vi "RTM - Tx Create Channels.vi"(6 "NumberOfInstances":u32, 7 "AppendToChannels":bool, 8 "error in (no error)":errorcluster, 9 "Descriptions":string[](array[string]), 10 "Channel Configuration":string[][](array[string]), 11 "Node Ptr":T1 format="%.0x") -> (0 "error out":errorcluster, 1 "ChannelPaths":string[](array[string]), 2 "ChannelNames":string[](array[string]), 4 "ChannelDataTypes":string[](array[string]), 5 "ChannelRefs":T1[](array[typedef]) format="%.0x")   [LabVIEW 2019, in "UDP-Custom-Device System Explorer.lvlib"]
uses:
  UDP-Custom-Device System Explorer.lvlib
  <vilib>/NI VeriStand/Custom Device API/Custom Device Item Ref.ctl
  <vilib>/NI VeriStand/Custom Device API/Custom Device Channel.ctl
  <vilib>/NI VeriStand/Custom Device API/Custom Device Channel Type.ctl
  Shared/Constants.vi
  <vilib>/NI VeriStand/Custom Device API/Custom Device API.lvlib
  Shared/UDP-Custom-Device Shared.lvlib
  Property Accessors/Tx Channel Section Accessors.lvlib
  Property Accessors/Tx Channel Accessors.lvlib
panel:
  out "ExistingChannels":string[](array[string])
  out "Dependent Node Refs":T1[](array[typedef]) format="%.0x"
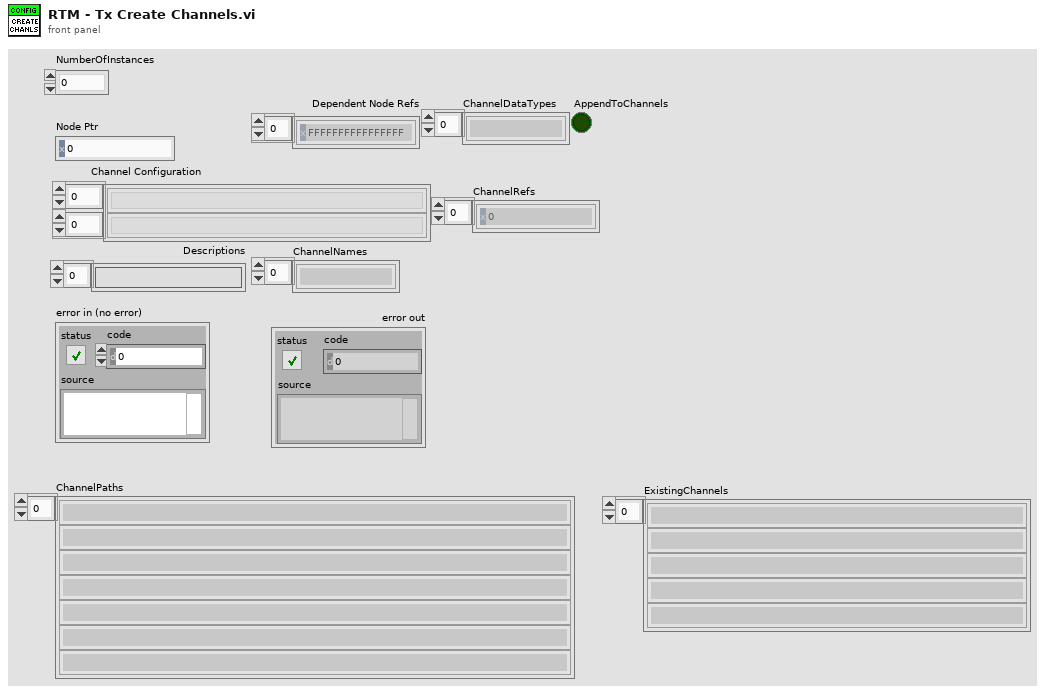
[diagram p1: front panel]
types:
  T1 = typedef "Custom Device API.lvlib/Custom Device Item Ref.ctl" = u64
  T2 = typedef "Custom Device API.lvlib/Custom Device Channel.ctl" = cluster{"Type":T3, "Units":string, "Default Value":dbl, "Faultable":bool, "Scalable":bool}
  T3 = typedef "Custom Device API.lvlib/Custom Device Channel Type.ctl" = enum16{"Input", "Output"}
  T4 = typedef "UDP-Custom-Device Shared.lvlib/Shared - Channel Data Type.ctl" = enum16{"Boolean", "Single", "Double", "I8", "I16", "I32", "I64", "U8", "U16", "U32", "U64"}
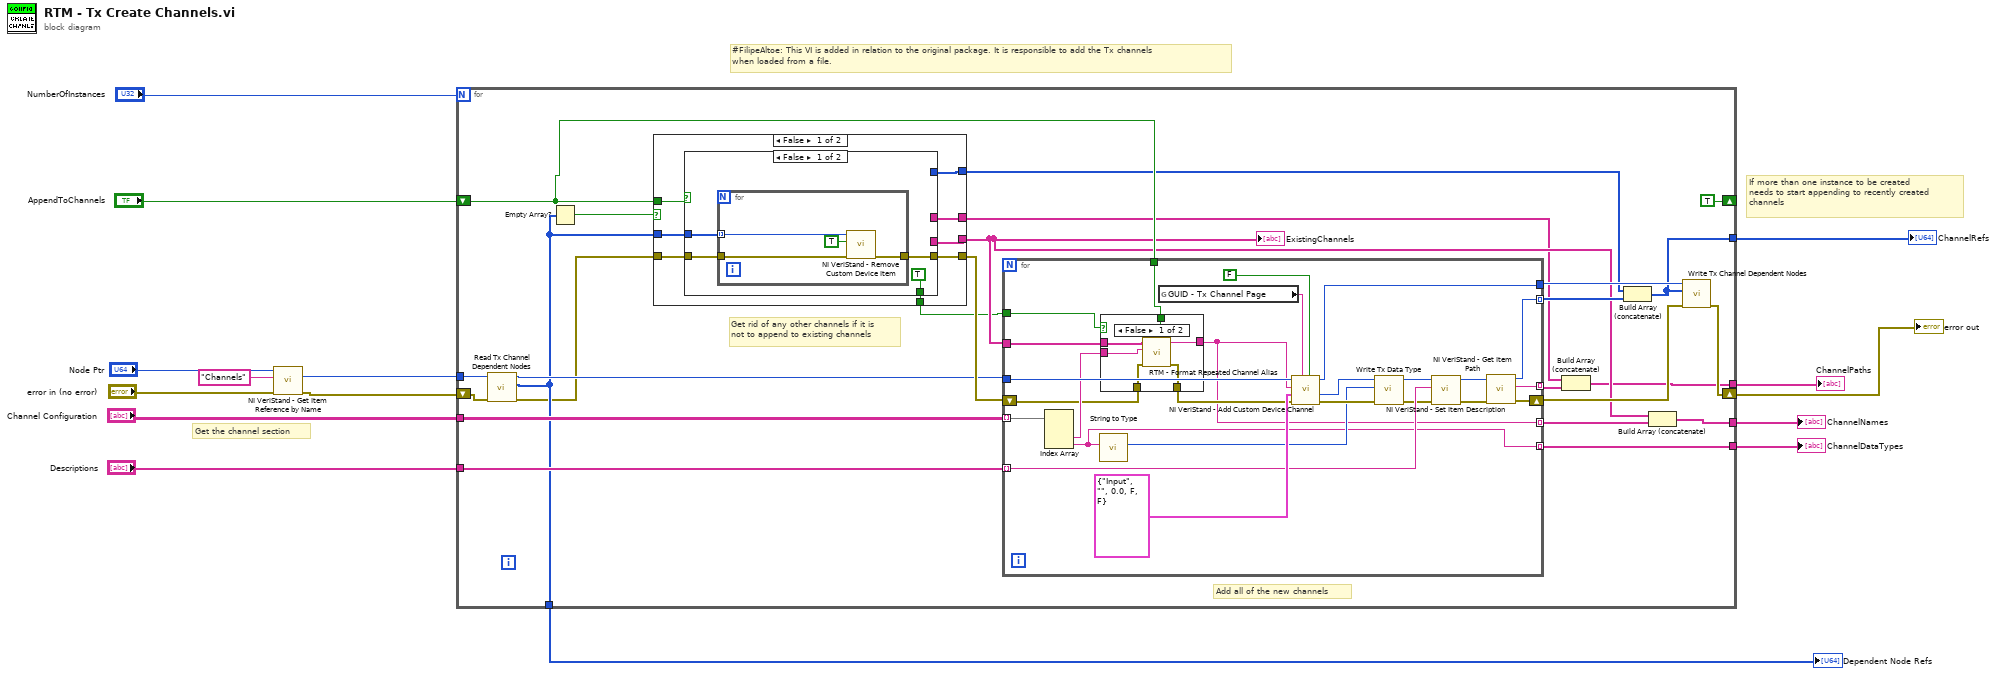
[diagram p0: block diagram]
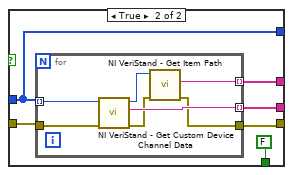
[diagram p3: hidden frame]
diagram:
  # "If more than one instance to be created\nneeds to start appending to recently created\nchannels"
  # "#FilipeAltoe: This VI is added in relation to the original package. It is responsible to add the Tx channels\nwhen loaded from a file."
  # "Get the channel section"
  n1 = call <vilib>:"NI VeriStand - Get Item Reference by Name.vi"("error in (no error)"="error in (no error)", "Item Name"="Channels" ("Section Name"), "Parent Ref in"="Node Ptr") -> ("error out"=w9:errorcluster, "Item Ref"=w3:T1)  [unwired: 5 in, 2 out]
  n2 = for {
    N: "NumberOfInstances" -> [_]
    tunnel: "Descriptions" -> [w39]
    tunnel: "Channel Configuration" -> [w38]
    tunnel: [w36] -> w10
    tunnel: [w25] -> w8
    tunnel: [w22] -> w6
    tunnel: [w18] -> w5
    tunnel: [w20] -> w4
    tunnel: w3 -> [w27]
    shift-right: [w31] -> w7
    shift-left: w9 -> [w35]
    shift-right: [TRUE ("AppendToChannels")] -> _
    shift-left: "AppendToChannels" -> [w26]
    # "Add all of the new channels"
    # "Get rid of any other channels if it is\nnot to append to existing channels"
    n3 = call "Read Tx Channel Dependent Nodes.vi"("error in (no error)"=w35, "Node Ptr"=w27) -> ("error out"=w34:errorcluster, "Dependent Node Refs"=w36:T1[], "Node Ptr out"=w37:T1)  [unwired: 7 in]
    n4 = Empty Array?(array=w36) -> (empty?=w23:bool)
    n5 = case shown="False" w23 {
      selector: w23 -> [_ w103]
      tunnel: [w81 w104] -> w40
      tunnel: w34 -> [w80 w104]
      tunnel: w36 -> [w79 _]
      tunnel: [w77 _] -> w21
      tunnel: w26 -> [w78 _]
      tunnel: [w76 _] -> w24
      tunnel: [w75 _] -> w19
      tunnel: [w74 w103] -> w17
      frame False {
        n6 = case shown="False" w78 {
          tunnel: [w85 w93] -> w81
          tunnel: w80 -> [w84 w95]
          tunnel: w79 -> [w83 w92]
          tunnel: [_ w94] -> w77
          tunnel: [_ w92] -> w76
          tunnel: [_ w91] -> w75
          tunnel: [TRUE FALSE] -> w74
          frame False {
            n7 = for {
              tunnel: w83 -> [w86] mode=indexing
              tunnel: [w88] -> w85
              tunnel: w84 -> [w87]
              n8 = call <vilib>:"NI VeriStand - Remove Custom Device Item.vi"("error in (no error)"=w87, "Force Delete (F)"=TRUE, "Item Ref in"=w86) -> ("error out"=w88:errorcluster)  [unwired: 7 in, 1 out]
            }
          }
          frame True {
            n9 = for {
              tunnel: w92 -> [w102] mode=indexing
              tunnel: [w98] -> w93
              tunnel: w95 -> [w101]
              tunnel: [w100] -> w94 mode=indexing
              tunnel: [w96] -> w91 mode=indexing
              n10 = call <vilib>:"NI VeriStand - Get Custom Device Channel Data.vi"("error in (no error)"=w101, "Channel Ref in"=w102) -> ("error out"=w99:errorcluster, "Channel Name"=w100:string, "Channel Ref out"=w97:T1)  [unwired: 4 in, 3 out]
              n11 = call <vilib>:"NI VeriStand - Get Item Path.vi"("error in (no error)"=w99, "Item Ref in"=w97) -> ("error out"=w98:errorcluster, "Path"=w96:string)  [unwired: 6 in, 2 out]
            }
          }
        }
      }
      frame True {
      }
    }
    "ExistingChannels" <- w21
    n12 = for {
      tunnel: w37 -> [w63]
      tunnel: w38 -> [w61] mode=indexing
      tunnel: w39 -> [w60] mode=indexing
      shift-right: [w50] -> w30
      shift-left: w40 -> [w45]
      tunnel: [w48] -> w32 mode=indexing
      tunnel: [w59] -> w33
      tunnel: [w42] -> w29 mode=indexing
      tunnel: [w53] -> w18 mode=indexing
      tunnel: [w49] -> w28 mode=indexing
      tunnel: w21 -> [w47]
      tunnel: w26 -> [w43]
      tunnel: w17 -> [w41]
      n13 = Index Array(array=w61) -> (element #2=w46:string, element #3=w53:string)  [unwired: 3 in, 1 out]
      n14 = call "String to Type.vi"("String Type"=w53) -> ("Data Type"=w56:T4)  [unwired: 10 in]
      n15 = case shown="False" w41 {
        tunnel: w47 -> [w71 _]
        tunnel: w46 -> [w70 w72]
        tunnel: w45 -> [w69 w73]
        tunnel: [w68 w73] -> w44
        tunnel: w43 -> [w67 _]
        tunnel: [w66 w72] -> w42
        frame False {
          n16 = call "RTM - Format Repeated Channel Alias.vi"("AppendToChannels"=w67, "error in (no error)"=w69, "ChannelName"=w70, "ExistingChannelNames"=w71) -> ("error out"=w68:errorcluster, "FormattedName"=w66:string)  [unwired: 6 in]
        }
        frame True {
        }
      }
      n17 = global read "Constants.vi" "GUID - Tx Channel Page"() -> (w64:string)
      n18 = call <vilib>:"NI VeriStand - Add Custom Device Channel.vi"("Highlight? (F)"=FALSE, "GUID (Default Channel)"=w64, "error in (no error)"=w44, "Channel"=T2 {"Type"=enum."Input", "Units"="", "Default Value"=0.0, "Faultable"=FALSE, "Scalable"=FALSE}, "Channel Name"=w42, "Parent Ref in"=w63) -> ("error out"=w58:errorcluster, "Channel Ref"=w57:T1, "Parent Ref out"=w59:T1)  [unwired: 2 in, 1 out]
      n19 = call "Write Tx Data Type.vi"("error in (no error)"=w58, "Data Type"=w56, "Node Ptr"=w57) -> ("error out"=w54:errorcluster, "Node Ptr out"=w55:T1)  [unwired: 6 in, 1 out]
      n20 = call <vilib>:"NI VeriStand - Set Item Description.vi"("error in (no error)"=w54, "Description"=w60, "Item Ref in"=w55) -> ("error out"=w52:errorcluster, "Item Ref out"=w51:T1)  [unwired: 6 in, 1 out]
      n21 = call <vilib>:"NI VeriStand - Get Item Path.vi"("error in (no error)"=w52, "Item Ref in"=w51) -> ("error out"=w50:errorcluster, "Path"=w49:string, "Item Ref out"=w48:T1)  [unwired: 6 in, 1 out]
    }
    n22 = Build Array (concatenate)(w19, w28) -> (w20:string[])
    n23 = Build Array (concatenate)(w24, w32) -> (w25:T1[])
    n24 = Build Array (concatenate)(w21, w29) -> (w22:string[])
    n25 = call "Write Tx Channel Dependent Nodes.vi"("error in (no error)"=w30, "Dependent Node Refs"=w25, "Node Ptr"=w33) -> ("error out"=w31:errorcluster)  [unwired: 7 in, 1 out]
  }
  "error out" <- w7
  "Dependent Node Refs" <- w10
  "ChannelNames" <- w6
  "ChannelDataTypes" <- w5
  "ChannelPaths" <- w4
  "ChannelRefs" <- w8
